vi "Flom Pump Control SubVI 01-13-11.vi"(1 "Flow Rate (uL)":dbl min=0.0 max=9900.0 step=1.0, 2 "Step #":i32=1 min=0 max=49 step=1, 3 "Time (.01 mins)":i32 min=0 max=9999 step=1, 4 "Stop   Start":bool=TRUE, 5 "Mode":string(combo)="Setup", 6 "Edit Values, or Run Flow?\n(Only for Continuous Flow)":string(combo), 7 "error in (no error)":errorcluster, 8 "Request Commands\n(Only for Status)":string(combo), 9 "Step Linear":bool=TRUE, 10 "Step Flow Commands \n(Only For Step Flow)":string(combo), 12 "Setup Commands\n(Only for Setup)":string(combo)) -> (14 "error out":errorcluster, 17 "String":string)   [LabVIEW 2015]
doc: "Use this template to parse data you acquired from an instrument and write the data to a file.\nNote: LabVIEW enables automatic error handling by default for VIs you create from this template."
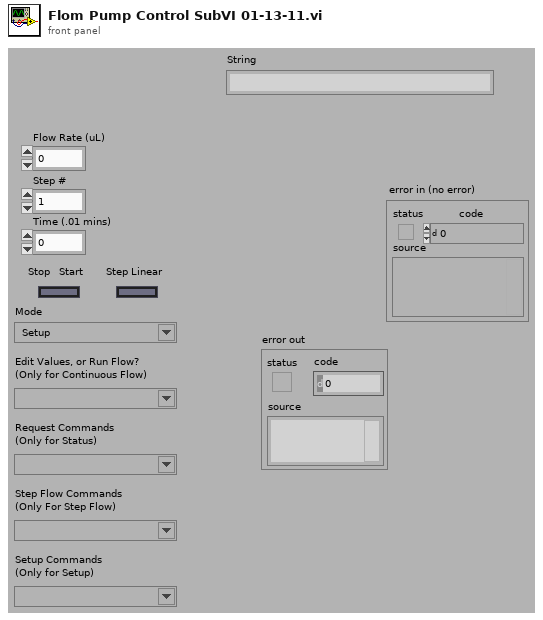
[diagram p1: front panel]
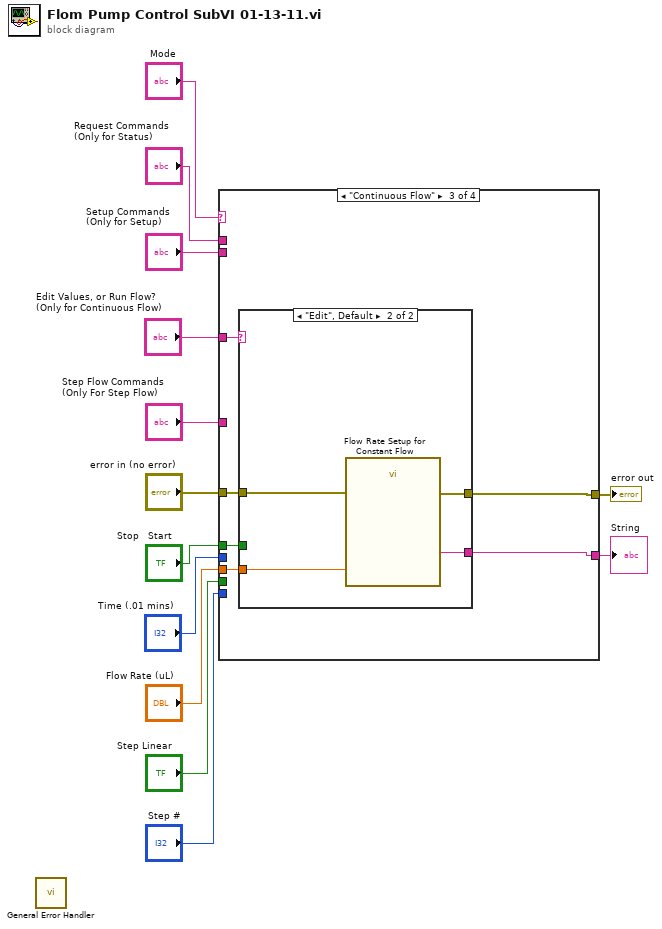
[diagram p0: block diagram]
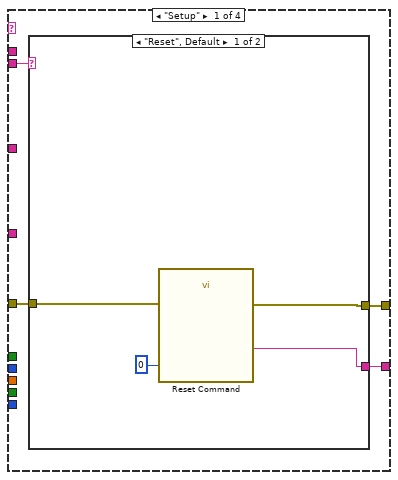
[diagram p2: hidden frame]
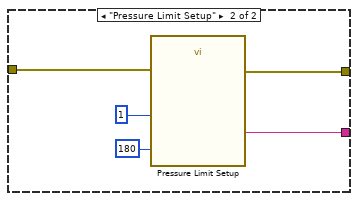
[diagram p3: hidden frame]
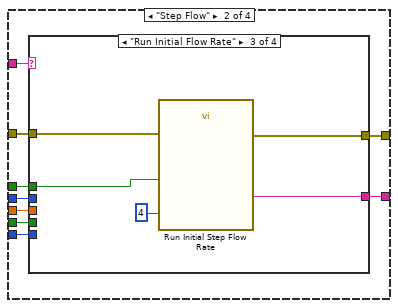
[diagram p4: hidden frame]
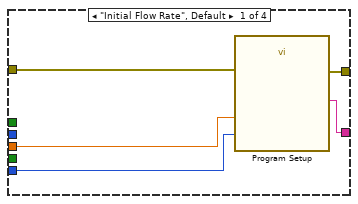
[diagram p5: hidden frame]
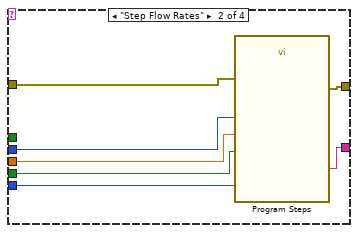
[diagram p6: hidden frame]
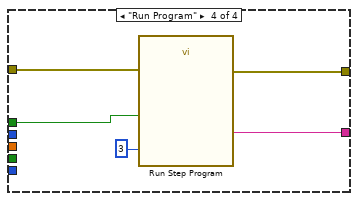
[diagram p7: hidden frame]
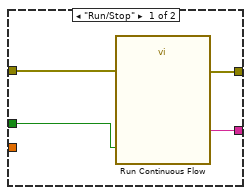
[diagram p8: hidden frame]
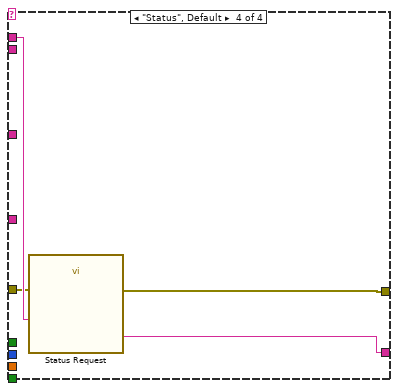
[diagram p9: hidden frame]
diagram:
  n1 = call <vilib>:"General Error Handler.vi"() -> ()  [unwired: 3 in, 13 out]
  n2 = case shown="\"Continuous Flow\"" "Mode" {
    tunnel: "Request Commands\n(Only for Status)" -> [_ _ _ w73]
    tunnel: "Setup Commands\n(Only for Setup)" -> [w17 _ _ _]
    tunnel: "Edit Values, or Run Flow?\n(Only for Continuous Flow)" -> [_ _ w63 _]
    tunnel: "Flow Rate (uL)" -> [_ w33 w62 _]
    tunnel: "Stop   Start" -> [_ w30 w61 _]
    tunnel: [w16 w35 w60 w75] -> w12
    tunnel: "Step #" -> [_ w34 _ _]
    tunnel: "Time (.01 mins)" -> [_ w32 _ _]
    tunnel: "Step Flow Commands \n(Only For Step Flow)" -> [_ w31 _ _]
    tunnel: [w15 w29 w59 w74] -> w13
    tunnel: "Step Linear" -> [_ w28 _ _]
    tunnel: "error in (no error)" -> [w14 w27 w58 w72]
    frame "Setup" {
      n3 = case shown="\"Reset\", Default" w17 {
        tunnel: [w21 w26] -> w16
        tunnel: [w20 w25] -> w15
        tunnel: w14 -> [w18 w22]
        frame "Reset", Default {
          n4 = call "Reset Command"("reset command"=0, "error in (no error)"=w18) -> ("Result"=w21:string, "error out"=w20:errorcluster)  [unwired: 2 in, 10 out]
        }
        frame "Pressure Limit Setup" {
          n5 = call "Pressure Limit Setup"("U Lim (0.1MPa)"=180, "L Lim (0.1MPa)"=1, "error in (no error)"=w22) -> ("Result"=w26:string, "error out"=w25:errorcluster)  [unwired: 2 in, 9 out]
        }
      }
    }
    frame "Step Flow" {
      n6 = case shown="\"Run Initial Flow Rate\"" w31 {
        tunnel: [w40 w47 w52 w57] -> w35
        tunnel: w34 -> [w38 w44 _ _]
        tunnel: w33 -> [w37 w43 _ _]
        tunnel: w32 -> [_ w45 _ _]
        tunnel: w30 -> [_ _ w49 w55]
        tunnel: [w39 w46 w51 w56] -> w29
        tunnel: w28 -> [_ w42 _ _]
        tunnel: w27 -> [w36 w41 w48 w53]
        frame "Initial Flow Rate", Default {
          n7 = call "Program Setup"("Number of Steps"=w38, "Stepped Initial Flow Rate"=w37, "error in (no error)"=w36) -> ("Result"=w40:string, "error out"=w39:errorcluster)  [unwired: 2 in, 9 out]
        }
        frame "Step Flow Rates" {
          n8 = call "Program Steps"("curve"=w42, "step number"=w44, "time .01 mins"=w45, "flow rate"=w43, "error in (no error)"=w41) -> ("Result"=w47:string, "error out"=w46:errorcluster)  [unwired: 1 in, 8 out]
        }
        frame "Run Initial Flow Rate" {
          n9 = call "Run Initial Step Flow Rate"("Flow mode"=4, "Start/Stop"=w49, "error in (no error)"=w48) -> ("Result"=w52:string, "error out"=w51:errorcluster)  [unwired: 2 in, 9 out]
        }
        frame "Run Program" {
          n10 = call "Run Step Program"("Flow mode"=3, "Start/Stop"=w55, "error in (no error)"=w53) -> ("Result"=w57:string, "error out"=w56:errorcluster)  [unwired: 2 in, 9 out]
        }
      }
    }
    frame "Continuous Flow" {
      n11 = case shown="\"Edit\", Default" w63 {
        tunnel: w62 -> [_ w69]
        tunnel: w61 -> [w65 _]
        tunnel: [w67 w71] -> w60
        tunnel: [w66 w70] -> w59
        tunnel: w58 -> [w64 w68]
        frame "Run/Stop" {
          n12 = call "Run Continuous Flow"("Start/Stop"=w65, "error in (no error)"=w64) -> ("Result"=w67:string, "error out"=w66:errorcluster)  [unwired: 2 in, 10 out]
        }
        frame "Edit", Default {
          n13 = call "Flow Rate Setup for Constant Flow"("flow rate in uL"=w69, "error in (no error)"=w68) -> ("Result"=w71:string, "error out"=w70:errorcluster)  [unwired: 2 in, 10 out]
        }
      }
    }
    frame "Status", Default {
      n14 = call "Status Request"("query"=w73, "error in (no error)"=w72) -> ("Result"=w75:string, "error out"=w74:errorcluster)  [unwired: 2 in, 10 out]
    }
  }
  "error out" <- w13
  "String" <- w12
